vi "Flip States.vi"(8 "error in (no error)":errorcluster, 11 "Flip States in":refnum<class "Flip States.lvclass">) -> (0 "error out":errorcluster, 3 "Flip States out":refnum<class "Flip States.lvclass">)   [LabVIEW 2021, in "Flip States.lvlib" / "Flip States.lvclass"]
uses:
  Flip States.lvclass
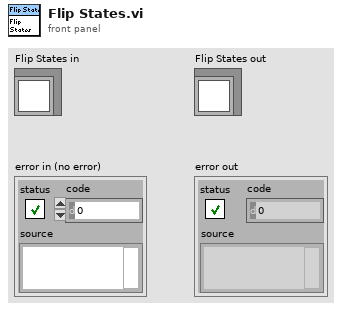
[diagram p1: front panel]
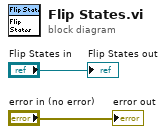
[diagram p0: block diagram]
diagram:
  "error out" <- "error in (no error)"
  "Flip States out" <- "Flip States in"
